vi "test2.vi"() -> ()   [LabVIEW 2013]
uses:
  VIs/ClientServerMode/CS_LFAClassGlobal.vi
  LightField Automation.lvclass
panel:
  in  "On Chip Accumulations 2":i32
  out "On Chip Accumulations":i32
  in  "Intensifier Gain":i32=1
  in  "?":bool
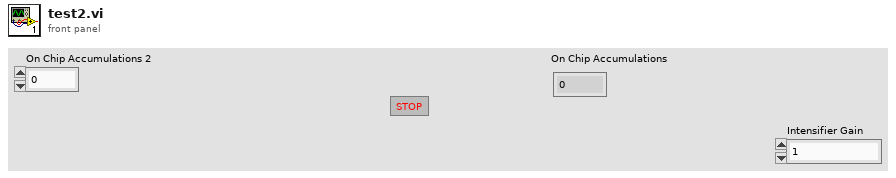
[diagram p1: front panel]
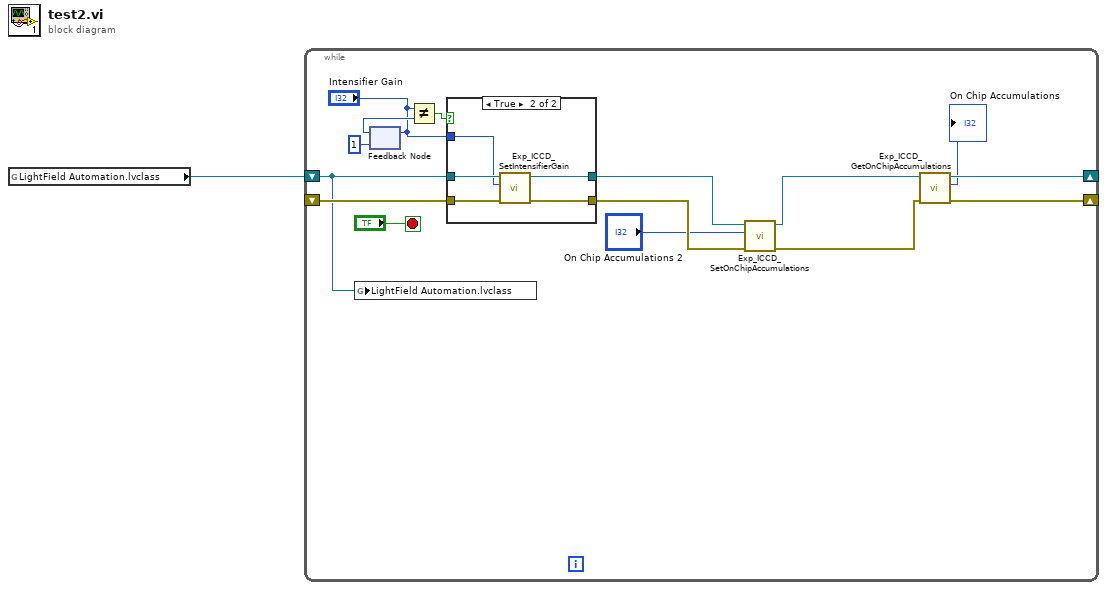
[diagram p0: block diagram]
diagram:
  n1 = global read "CS_LFAClassGlobal.vi" "LightField Automation.lvclass"() -> (w1:refnum<class "LightField Automation.lvclass">)
  n2 = while {
    shift-right: [w9] -> _
    shift-left: w1 -> [w2]
    shift-right: [w10] -> _
    shift-left: _ -> [w13]
    stop <- "?" stop-if-true
    n3 = global write "CS_LFAClassGlobal.vi" "LightField Automation.lvclass"(w2) -> ()
    n4 = feedback #1(1 ("Intensifier Gain")) -> (w15:i32)
    n5 = feedback-in #1("Intensifier Gain") -> ()
    n6 = Not Equal?(x="Intensifier Gain", y=w15) -> (x != y?=w14:bool)
    n7 = case shown="True" w14 {
      tunnel: "Intensifier Gain" -> [_ w19]
      tunnel: w2 -> [w17 w23]
      tunnel: w13 -> [w18 w22]
      tunnel: [w17 w20] -> w7
      tunnel: [w18 w21] -> w6
      frame False {
      }
      frame True {
        n8 = call "Exp_ICCD_SetIntensifierGain.vi"("error in (no error)"=w22, "Intensifier Gain"=w19, "LightField Automation in"=w23) -> ("error out"=w21:errorcluster, "LightField Automation out"=w20:refnum<class "LightField Automation.lvclass">)  [unwired: 7 in]
      }
    }
    n9 = call "Exp_ICCD_SetOnChipAccumulations.vi"("error in (no error)"=w6, "On Chip Accumulations"="On Chip Accumulations 2", "LightField Automation in"=w7) -> ("error out"=w4:errorcluster, "LightField Automation out"=w5:refnum<class "LightField Automation.lvclass">)  [unwired: 7 in]
    n10 = call "Exp_ICCD_GetOnChipAccumulations.vi"("error in (no error)"=w4, "LightField Automation in"=w5) -> ("error out"=w10:errorcluster, "On Chip Accumulations"=→"On Chip Accumulations":i32, "LightField Automation out"=w9:refnum<class "LightField Automation.lvclass">)  [unwired: 7 in]
  }
